vi "niFpgaWriteControlTemplate.vi"(0 "reference":refnum<vi>, 5 "Control Name":string, 7 "Value":variant, 11 "error in (no error)":errorcluster) -> (15 "error out":errorcluster)   [LabVIEW 2017]
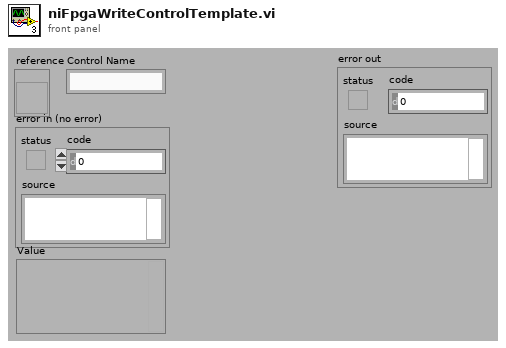
[diagram p1: front panel]
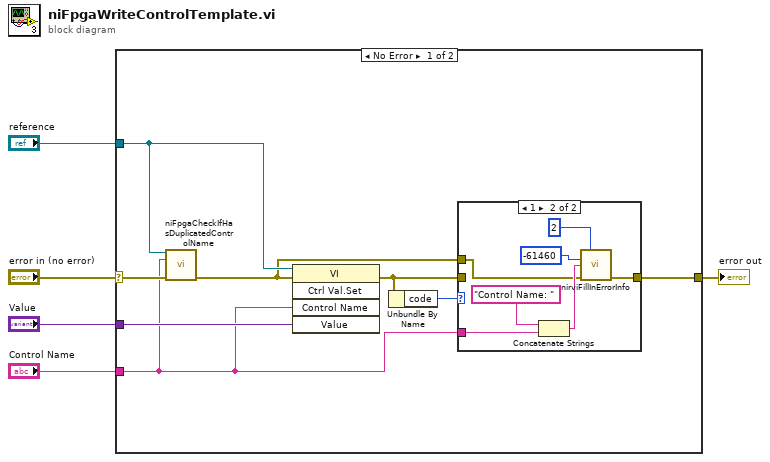
[diagram p0: block diagram]
diagram:
  n1 = case shown="No Error" "error in (no error)" {
    selector: "error in (no error)" -> [w9 w22]
    tunnel: "reference" -> [w8 _]
    tunnel: "Value" -> [w13 _]
    tunnel: [w12 w22] -> w3
    tunnel: "Control Name" -> [w6 _]
    frame No Error {
      n2 = call <vilib>:"niFpgaCheckIfHasDuplicatedControlName.vi"("reference"=w8, "Control Name"=w6, "error in (no error)"=w9) -> ("error out"=w7:errorcluster)  [unwired: 12 in]
      n3 = invoke class="VI" method="Ctrl Val.Set"(reference=w8, error in=w7, "Control Name"=w6, "Value"=w13) -> (error out=w10:errorcluster)  [unwired: 1 in, 4 out]
      n4 = Unbundle By Name(w10) -> ("code"=w11:i32)
      n5 = case shown="1" w11 {
        tunnel: w10 -> [w14 _]
        tunnel: [w14 w21] -> w12
        tunnel: w6 -> [_ w18]
        tunnel: w7 -> [_ w16]
        frame Default {
        }
        frame 1 {
          n6 = Concatenate Strings("Control Name: " ("extended error info"), w18) -> (w17:string)
          n7 = call <vilib>:"nirviFillInErrorInfo.vi"("depth"=2, "status code"=-61460, "extended error info"=w17, "error in"=w16) -> ("error out"=w21:errorcluster)  [unwired: 11 out]
        }
      }
    }
    frame Error {
    }
  }
  "error out" <- w3
